vi "Launch Nested Digital Reader Actor.vi"(8 "error in (no error)":errorcluster, 10 "Nested Digital Reader Actor":refnum<class "Digital Reader.lvclass">, 11 "Caller Actor in":refnum<class "Actor.lvclass">) -> (3 "Caller Actor out":refnum<class "Actor.lvclass">)   [LabVIEW 2024, in "DAQmx Actor.lvlib" / "Digital Reader.lvclass"]
uses:
  Digital Reader.lvclass
  Digital Reader.lvclass/Digital Reader.ctl
  <vilib>/ActorFramework/Actor/Actor.lvclass
  C:/Users/uspoaotto/OneDrive - Oregon Tool/Desktop/working copies/DAQmxActor/src/DAQmx Actor/DAQmx Actor/DAQmx Actor.lvclass
  C:/Program Files (x86)/National Instruments/LabVIEW 2024/vi.lib/ActorFramework/Actor/Actor.lvclass
  C:/Users/uspoaotto/OneDrive - Oregon Tool/Desktop/working copies/DAQmxActor/src/DAQmx Actor/Digital Reader/Digital Reader.lvclass
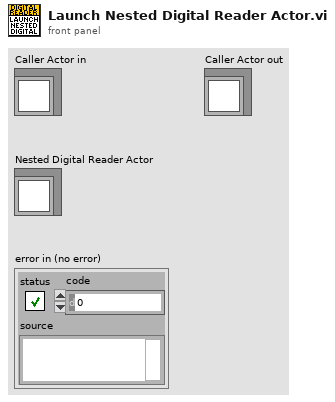
[diagram p1: front panel]
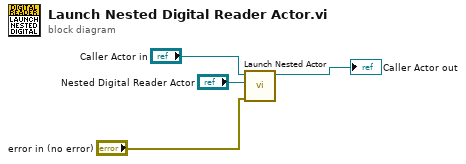
[diagram p0: block diagram]
diagram:
  n1 = call <vilib>:"Launch Nested Actor.vi"("error in (no error)"="error in (no error)", "Nested Actor"="Nested Digital Reader Actor", "Caller Actor in"="Caller Actor in") -> ("Caller Actor out"=→"Caller Actor out":refnum<class "Actor.lvclass">)  [unwired: 6 in, 2 out]
